vi "New Session ID.vi"(8 "error in (no error)":errorcluster, 11 "object in":refnum<class "JuPyter_Client.lvclass">) -> (0 "error out":errorcluster, 3 "object out":refnum<class "JuPyter_Client.lvclass">)   [LabVIEW 2018, in "JuPyter_Client.lvclass"]
doc: "Create a new session ID and rest message counter"
uses:
  JuPyter_Client.lvclass
  JuPyter_Client.lvclass/JuPyter_Client.ctl
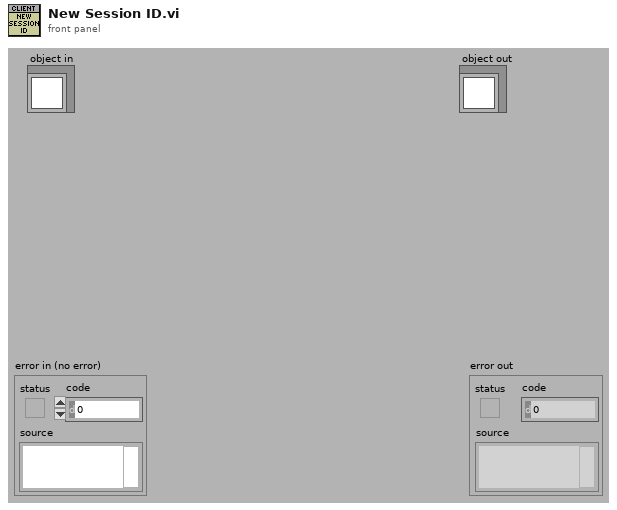
[diagram p1: front panel]
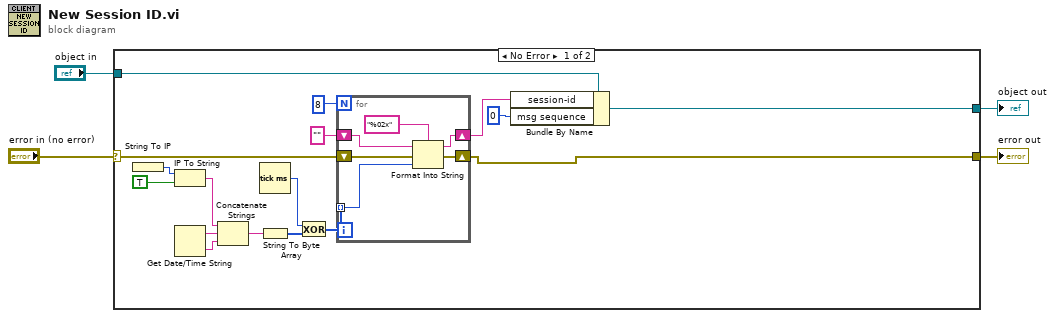
[diagram p0: block diagram]
diagram:
  n1 = case shown="No Error" "error in (no error)" {
    selector: "error in (no error)" -> [w12 w29]
    tunnel: [w5 w29] -> w3
    tunnel: [w6 w28] -> w1
    tunnel: "object in" -> [w21 w28]
    frame No Error {
      n2 = String To IP() -> (0:w20:u32)  [unwired: 1 in]
      n3 = IP To String(1:TRUE ("dot notation? (F)"), 2:w20) -> (0:w18:string)
      n4 = Get Date/Time String() -> (date string=w17:string, time string=w16:string)  [unwired: 3 in]
      n5 = Concatenate Strings(w18, w17, w16) -> (w15:string)
      n6 = Tick Count (ms)() -> (millisecond timer value=w9:u32)
      n7 = String To Byte Array(string=w15) -> (unsigned byte array=w13:u8[])
      n8 = Exclusive Or(1:w13, 2:w9) -> (0:w10:u32[])
      n9 = for {
        N: 8 -> [_]
        tunnel: w10 -> [w27] mode=indexing
        shift-right: [w26] -> w7
        shift-left: "" -> [w25]
        shift-right: [w23] -> w5
        shift-left: w12 -> [w22]
        n10 = Format Into String(format string="%02x", initial string=w25, error in=w22, w27) -> (resulting string=w26:string, error out=w23:errorcluster)
      }
      n11 = Bundle By Name(cluster=w21, "session-id"=w7, "msg sequence"=u64 0) -> (w6:refnum<class "JuPyter_Client.lvclass">)
    }
    frame Error {
    }
  }
  "error out" <- w3
  "object out" <- w1
